vi "Multimeter_Reset.vi"(8 "error in (no error)":errorcluster, 11 "MultimeterControl in":refnum<class "MultimeterControl.lvclass">) -> (0 "error out":errorcluster, 3 "MultimeterControl out":refnum<class "MultimeterControl.lvclass">)   [LabVIEW 2018, in "MultimeterControl.lvclass"]
uses:
  MultimeterControl.lvclass
  C:/Users/itk/Documents/itk-strip-sensor-qc/InstrControl/InstrControl.lvclass
  InstrControl.lvclass
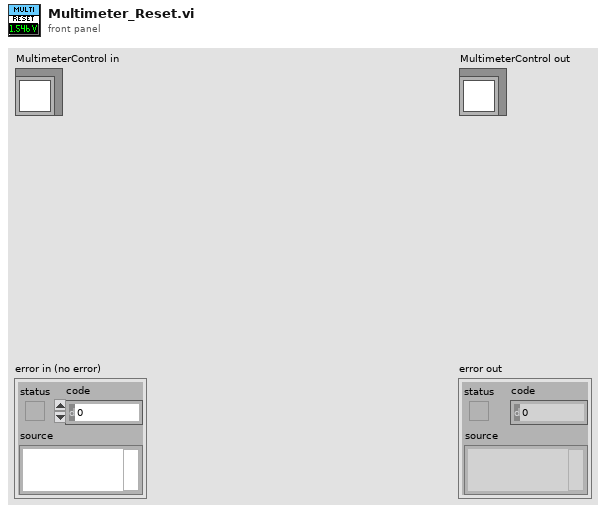
[diagram p1: front panel]
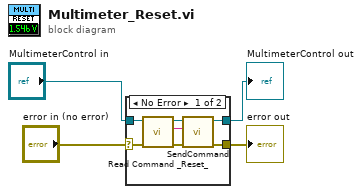
[diagram p0: block diagram]
diagram:
  n1 = case shown="No Error" "error in (no error)" {
    selector: "error in (no error)" -> [w10 w13]
    tunnel: [w8 w13] -> w3
    tunnel: [w6 w12] -> w1
    tunnel: "MultimeterControl in" -> [w11 w12]
    frame No Error {
      n2 = call-dynamic "Read Command _Reset_.vi"("error in (no error)"=w10, "MultimeterControl in"=w11) -> ("error out"=w9:errorcluster, "Command \"Reset\""=w5:string, "MultimeterControl out"=w7:refnum<class "MultimeterControl.lvclass">)  [unwired: 7 in]
      n3 = call "SendCommand.vi"("error in (no error)"=w9, "Command string"=w5, "InstControl in"=w7) -> ("error out"=w8:errorcluster, "InstControl out"=w6:refnum<class "MultimeterControl.lvclass">)  [unwired: 7 in]
    }
    frame Error {
    }
  }
  "error out" <- w3
  "MultimeterControl out" <- w1
